vi "op-read.vi"(0 "Chain IN":bool) -> (1 "Moving Left Drive":bool, 2 "Moving Right Drive":bool, 3 "Moving Arm":bool, 4 "Chain OUT":bool, 6 "Encoder Left Drive":dbl, 8 "Encoder Right Drive":dbl, 10 "Encoder Arm":dbl)   [LabVIEW 2010, in "LASA Beta.lvrbt"]
uses:
  LASA Beta.lvrbt
  <vilib>/NXT/NXTIO Xnodes/AddressXNode/NXTIOAddress.xnode
  <vilib>/NXT/Subs/MotorXNode.DC Motor Type.ctl
  <vilib>/NXT/Subs/MotorXNode.1DCMotor.ctl
  <vilib>/NXT/Subs/MotorXNode.2DCMotor.ctl
  <vilib>/NXT/Subs/LVHSConnector.ctl
  <vilib>/NXT/NXTIO Xnodes/NXTIOXNode/NXTIO.xnode
  <vilib>/NXT/NXTIO Xnodes/NXTIONodeSubVIs/TETRIX IO Motor Status.vi
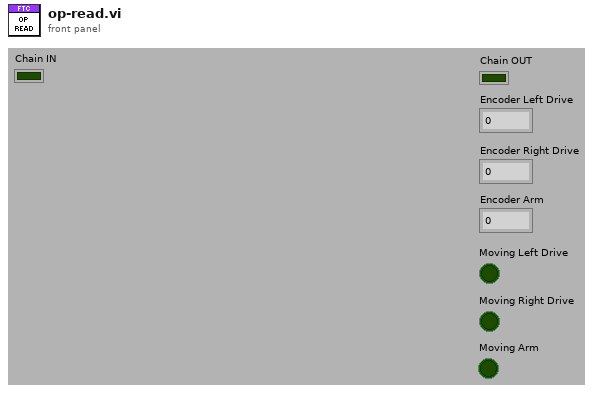
[diagram p1: front panel]
types:
  T1 = typedef "MotorXNode.DC Motor Type.ctl" = enum16{"DC Motor"}
  T2 = cluster{"DC Motor":T1, "Address":i16, "Address":i16}
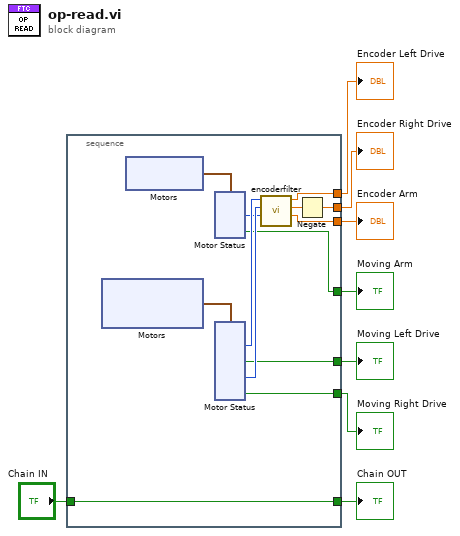
[diagram p0: block diagram]
diagram:
  n1 = stacked-sequence {
    tunnel: [w15] -> w8
    tunnel: [w14] -> w7
    tunnel: [w13] -> w6
    tunnel: [w12] -> w5
    tunnel: [w11] -> w4
    tunnel: [w10] -> w3
    tunnel: [w9] -> w2
    tunnel: "Chain IN" -> [w9]
    frame #0 {
      n2 = xnode "Motors"() -> ("DC Motor"=w21:T2)
      n3 = xnode "Motors"() -> ("DC Motor"=w19:cluster{"DC Motor":T1, "Address":i16})
      n4 = xnode "Motor Status"("Motors"=w19) -> ("Moving 1"=w12:bool, "Position 1"=w16:i32)  [unwired: 1 in, 1 out]
      n5 = xnode "Motor Status"("Motors"=w21) -> ("Moving 2"=w10:bool, "Moving 1"=w11:bool, "Position 2"=w17:i32, "Position 1"=w18:i32)  [unwired: 1 in, 1 out]
      n6 = call "encoderfilter.vi"("Encoder Input 3"=w16, "Encoder Input 2"=w17, "Encoder Input"=w18) -> ("Encoder Output 3"=w13:dbl, "Encoder Output 2"=w20:dbl, "Encoder Output"=w14:dbl)  [unwired: 5 in, 1 out]
      n7 = Negate(x=w20) -> (-x=w15:dbl)
    }
  }
  "Chain OUT" <- w2
  "Encoder Left Drive" <- w7
  "Encoder Right Drive" <- w8
  "Moving Left Drive" <- w4
  "Moving Right Drive" <- w3
  "Moving Arm" <- w5
  "Encoder Arm" <- w6
